vi "niusrprios Rx Core.vi"(0 "ddc parameters":T1[](array[typedef])=[{"output sample rate"=0.0, "delay"=0.0, "frequency shift"=0.0, "impairments"={"inline gain I"=0.0, "inline gain Q"=0.0, "cross gain I"=0.0, "cross gain Q"=0.0, "pre-gain offset I"=0.0, "pre-gain offset Q"=0.0, "post-gain offset I"=0.0, "post-gain offset Q"=0.0}, "phase"=0.0}, {"output sample rate"=0.0, "delay"=0.0, "frequency shift"=0.0, "impairments"={"inline gain I"=0.0, "inline gain Q"=0.0, "cross gain I"=0.0, "cross gain Q"=0.0, "pre-gain offset I"=0.0, "pre-gain offset Q"=0.0, "post-gain offset I"=0.0, "post-gain offset Q"=0.0}, "phase"=0.0}] {"frequency shift" format="%#.48g"}, 1 "rx.reset":bool=TRUE, 5 "rx.samples to acquire":u32, 7 "rx.abort":bool, 9 "rx.stream enable":bool[](array[boolean])=[FALSE, FALSE], 11 "rx.start trigger":bool) -> (4 "rx.state":T3, 6 "rx.samples processed":u32, 8 "rx.number of fifo overflows":u32, 10 "rx 0.number of IQ data overflows":u64, 14 "rx.dsp reset done":bool, 15 "rx 1.number of IQ data overflows":u64)   [LabVIEW 2015]
uses:
  niusrprios Stream Control State.ctl
  niusrprios DDC Parameters.ctl
  <instrlib>/_niInstr/DSP/v1/Shared/Public/IQ Impairments.ctl
  <vilib>/rvi/eio/common/nirviEmuTemplateMethod_errors.vi
  <vilib>/eio/EIONode/EIONode.xnode
  <instrlib>/_niInstr/Basic Elements/v1/FPGA/niInstr Basic Elements v1 FPGA.lvlib
  <instrlib>/_niInstr/DSP/v1/FPGA/niInstr DSP v1 FPGA.lvlib
  <instrlib>/_niInstr/DSP/v1/Shared/niInstr DSP v1 Shared.lvlib
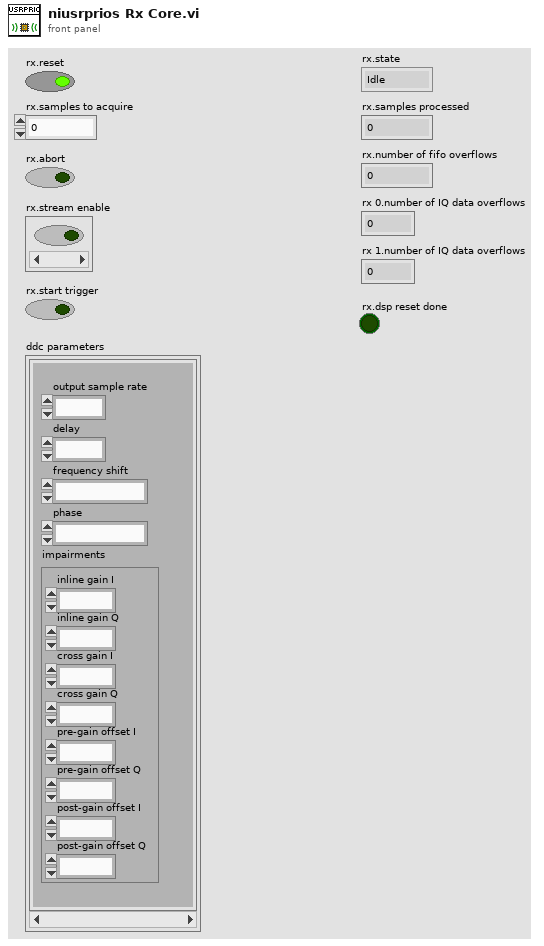
[diagram p1: front panel]
types:
  T1 = typedef "niusrprios DDC Parameters.ctl" = cluster{"output sample rate":fxp<+,48,1>, "delay":fxp<+/-,16,0>, "frequency shift":fxp<+/-,48,0>, "impairments":T2, "phase":fxp<+/-,21,0>}
  T2 = typedef "niInstr DSP v1 Shared.lvlib/IQ Impairments.ctl" = cluster{"inline gain I":fxp<+/-,18,1>, "inline gain Q":fxp<+/-,18,1>, "cross gain I":fxp<+/-,18,1>, "cross gain Q":fxp<+/-,18,1>, "pre-gain offset I":fxp<+/-,18,1>, "pre-gain offset Q":fxp<+/-,18,1>, "post-gain offset I":fxp<+/-,18,1>, "post-gain offset Q":fxp<+/-,18,1>}
  T3 = typedef "niusrprios Stream Control State.ctl" = enum16{"Idle", "Active"}
  T4 = typedef "niInstr DSP v1 Shared.lvlib/IQ Data.ctl" = cluster{"I":fxp<+/-,18,1>, "Q":fxp<+/-,18,1>, "overflow":bool}
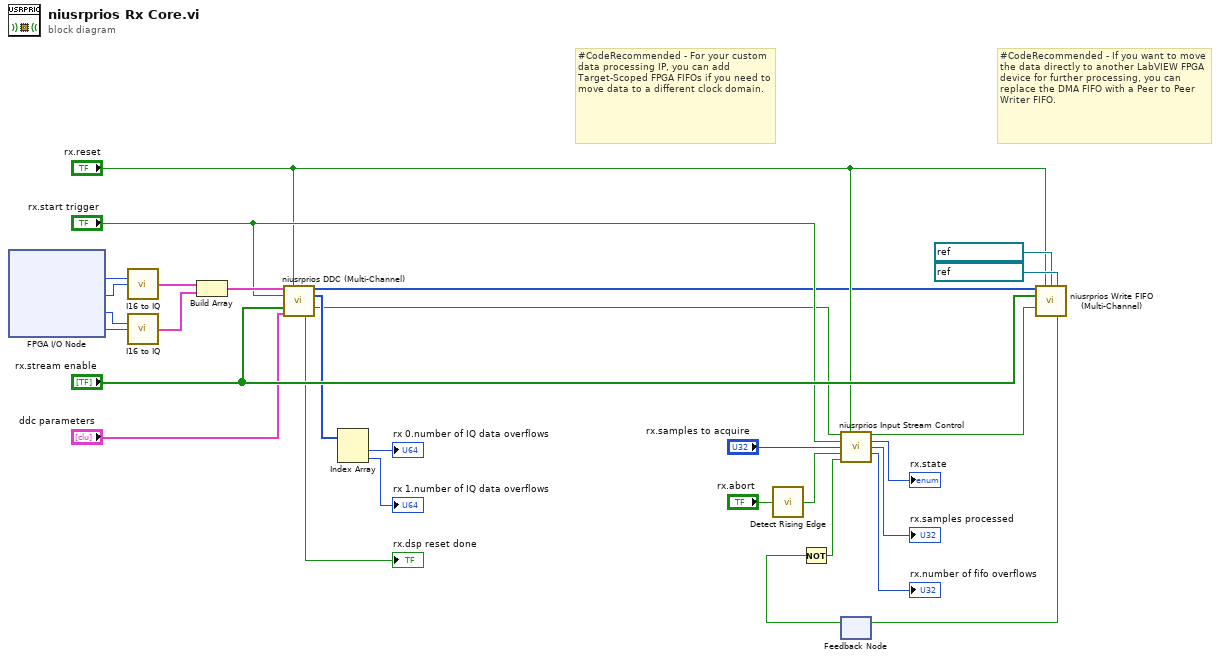
[diagram p0: block diagram]
diagram:
  # "#CodeRecommended - If you want to move the data directly to another LabVIEW FPGA device for further processing, you can replace the DMA FIFO with a Peer to Peer Writer FIFO."
  # "#CodeRecommended - For your custom data processing IP, you can add Target-Scoped FPGA FIFOs if you need to move data to a different clock domain."
  n1 = xnode "FPGA I/O Node"() -> ("RF 0/Rx/I"=w8:i16, "RF 0/Rx/Q"=w9:i16, "RF 1/Rx/I"=w21:i16, "RF 1/Rx/Q"=w22:i16)  [unwired: 4 in, 4 out]
  n2 = call <instrlib>:"I16 to IQ.vi"("I"=w8, "Q"=w9) -> ("IQ"=w10:T4)  [unwired: 13 in]
  n3 = call <instrlib>:"I16 to IQ.vi"("I"=w21, "Q"=w22) -> ("IQ"=w11:T4)  [unwired: 13 in]
  n4 = Build Array(w10, w11) -> (w28:T4[])
  n5 = call "niusrprios DDC (Multi-Channel).vi"("data in"=w28, "reset"="rx.reset", "start trigger"="rx.start trigger", "enabled"="rx.stream enable", "DDC Parameters"="ddc parameters") -> ("data out"=w15:u32[], "number of overflows"=w27:u64[], "output valid"=w25:bool, "dsp reset done"=→"rx.dsp reset done":bool)  [unwired: 7 in]
  n6 = Index Array(array=w27) -> (element #1=→"rx 0.number of IQ data overflows":u64, element #2=→"rx 1.number of IQ data overflows":u64)  [unwired: 2 in]
  n7 = call <instrlib>:"Detect Rising Edge.vi"("signal"="rx.abort") -> ("edge detected"=w7:bool)  [unwired: 14 in]
  n8 = feedback #1() -> (w14:bool)  [unwired: 1 in]
  n9 = Not(x=w14) -> (.not. x?=w4:bool)
  n10 = call "niusrprios Input Stream Control.vi"("input valid"=w25, "reset"="rx.reset", "start trigger"="rx.start trigger", "burst size"="rx.samples to acquire", "abort"=w7, "fifo timeout"=w4) -> ("write stream"=w23:bool, "state"=→"rx.state":T3, "samples processed"=→"rx.samples processed":u32, "number of overflows"=→"rx.number of fifo overflows":u32)  [unwired: 5 in, 1 out]
  n11 = call "niusrprios Write FIFO (Multi-Channel).vi"("data in"=w15, "reset"="rx.reset", "FIFO 0"=refnum<k21> "Rx Stream 0" ("fifo"), "FIFO 1"=refnum<k21> "Rx Stream 1" ("fifo"), "enabled"="rx.stream enable", "input valid"=w23) -> ("ready for input"=w17:bool)  [unwired: 9 in]
  n12 = feedback-in #1(w17) -> ()
